vi "Ceyear Acquire Trace.vi"() -> ()   [LabVIEW 2021]
doc: "This example shows how to configure the spectrum analyzer to acquire a trace."
uses:
  <instrlib>/Ceyear/Ceyear.lvlib
  <instrlib>/Ceyear/Public/Configure/Configure lbd (Center Span).vi
panel:
  out "Trace Waveform":T1(graph)
  in  "Manual Detector Type (0: Positive)":u16(ring) items=["Positive", "RMS", "Negative", "Sample"]
  in  "Reference Level Offset (0 dB)":dbl
  in  "Reference Level (10 dBm)":dbl=10.0
  in  "Input Impedance (0: 50 ohms)":u16(ring) items=["50", "75"]
  in  "Trace Type (0: Clear Write)":u16(ring) items=["Clear Write", "Maximum Hold", "Minimum Hold", "View"]
  in  "Stop Frequency (2 GHz)":dbl=2000000000.0
  in  "Start Frequency (0 Hz)":dbl
  in  "VISA resource name":refnum<visa-resource-name>
  # "(c) 2014 <Enter Company Name Here>.  ALL RIGHTS RESERVED."
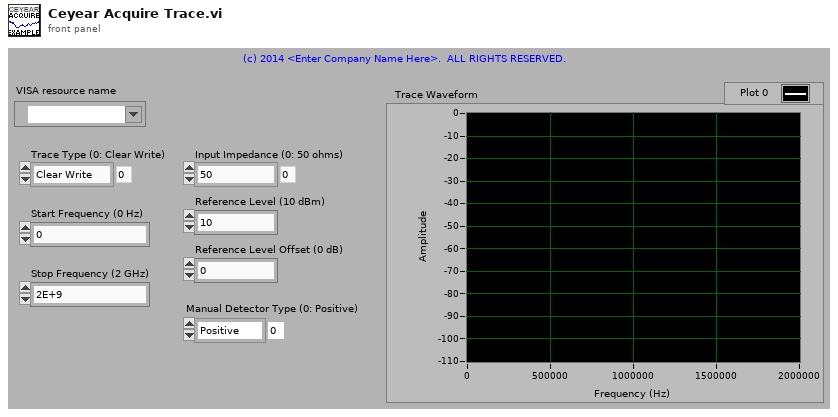
[diagram p1: front panel]
types:
  T1 = cluster{"Start Frequency (0 Hz)":dbl, dbl, "Trace":sgl[]}
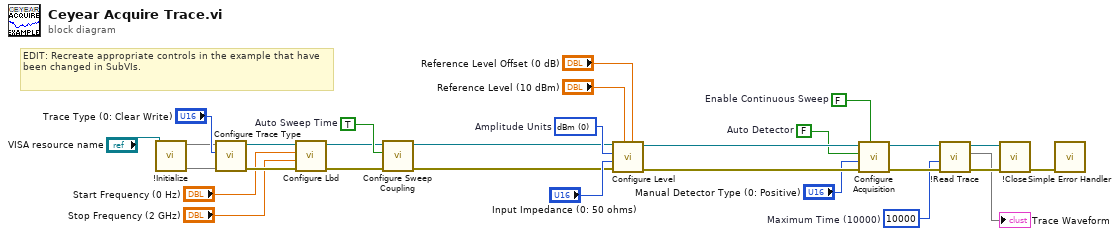
[diagram p0: block diagram]
diagram:
  w2 = u32 10000  # Maximum Time (10000)
  w11 = TRUE  # Auto Sweep Time
  w17 = FALSE  # Auto Detector
  w1 = FALSE  # Enable Continuous Sweep
  w21 = u16 0 items=["dBm", "dBV", "dBmV", "dBuV", "Volts", "Watts"]  # Amplitude Units
  # "EDIT: Recreate appropriate controls in the example that have been changed in SubVIs."
  n1 = call <instrlib>:"!Initialize.vi"(11:"VISA resource name") -> (0:w14, 3:w15)  [unwired: 9 in]
  n2 = call <instrlib>:"Configure Trace Type.vi"("error in (no error)"=w14, "Trace Type (0: Clear Write)"="Trace Type (0: Clear Write)", "VISA resource name"=w15) -> ("error out"=w5:errorcluster, "VISA resource name out"=w8:refnum<visa-resource-name>)  [unwired: 7 in]
  n3 = call-poly <instrlib>:"Configure Lbd.vi"("error in (no error)"=w5, "Span (0.1 - 1100 nm)"="Stop Frequency (2 GHz)", "Center lbd (600.05 - 1699.95 nm)"="Start Frequency (0 Hz)", "VISA resource name"=w8) -> ("error out"=w6:errorcluster, "VISA resource name out"=w7:refnum<visa-resource-name>)  [unwired: 6 in]
  n4 = call <instrlib>:"Configure Sweep Coupling.vi"("error in (no error)"=w6, "Auto Sweep Time (T: Enable)"=w11, "VISA resource name"=w7) -> ("error out"=w12:errorcluster, "VISA resource name out"=w13:refnum<visa-resource-name>)  [unwired: 7 in]
  n5 = call <instrlib>:"Configure Level.vi"("Reference Level Offset (0 dB)"="Reference Level Offset (0 dB)", "Reference Level (0)"="Reference Level (10 dBm)", "error in (no error)"=w12, "Input Impedance (0: 50 ohms)"="Input Impedance (0: 50 ohms)", "Amplitude Units (0: dBm)"=w21, "VISA resource name"=w13) -> ("error out"=w22:errorcluster, "VISA resource name out"=w23:refnum<visa-resource-name>)  [unwired: 4 in]
  n6 = call <instrlib>:"Configure Acquisition.vi"("Enable Continuous Sweep (F: Disable)"=w1, "error in (no error)"=w22, "Manual Detector Type (0: Positive)"="Manual Detector Type (0: Positive)", "Auto Detector (F: Disable)"=w17, "VISA resource name"=w23) -> ("error out"=w29:errorcluster, "VISA resource name out"=w28:refnum<visa-resource-name>)  [unwired: 5 in]
  n7 = call <instrlib>:"!Read Trace.vi"("error in (no error)"=w29, "Maximum Time (10000)"=w2, "VISA resource name"=w28) -> ("error out"=w25:errorcluster, 2:→"Trace Waveform", "VISA resource name out"=w27:refnum<visa-resource-name>)  [unwired: 6 in]
  n8 = call <instrlib>:"!Close.vi"("error in (no error)"=w25, "VISA resource name"=w27) -> ("error out"=w26:errorcluster)  [unwired: 9 in]
  n9 = call <vilib>:"Simple Error Handler.vi"("error in (no error)"=w26) -> ()  [unwired: 4 in, 5 out]
